vi "PFMate-Remote.vi"(2 "Channel":u8=1, 11 "Port":u8=1) -> ()   [LabVIEW 2009]
panel:
  in  "?":bool=TRUE
  in  "?":dbl(knob)=6.0 min=1.0 max=7.0 step=1.0 scale=1.0..7.0
  in  "?":dbl(knob)=5.0 min=1.0 max=7.0 step=1.0 scale=1.0..7.0
  in  "?":u8(ring)
  in  "?":u8(ring) items=["Run", "Float", "Brake"]
  in  "?":u8(ring) items=["Run", "Float", "Brake"]
  in  "?":bool=TRUE
  in  "PFMate address":u8=72 caption="PFMate Address" format="%x"
  # "Motor A"
  # "Motor B"
  # "mindsensors.com\nCopyright (c) 2009 by mindsensors.com\nEmail: info (<at>) mindsensors (<dot>) com\n\nThis program is free software. You can redistribute it and/or modify\nit under the terms of the GNU General Public License as published by\nthe Free Software Foundation; version 3 of the License.\nRead the license at: http://www.gnu.org/licenses/gpl.txt"
  # "Mode"
  # "Direction"
  # "Power"
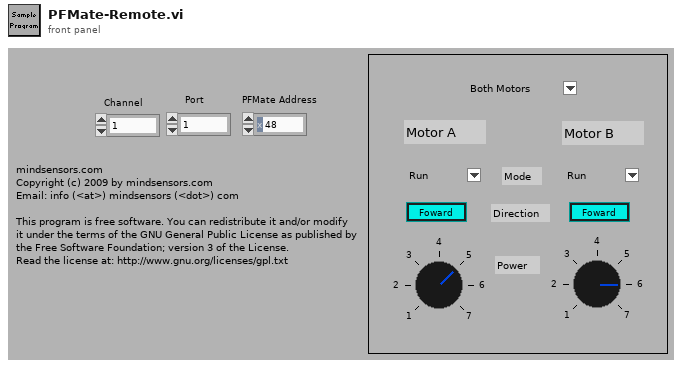
[diagram p1: front panel]
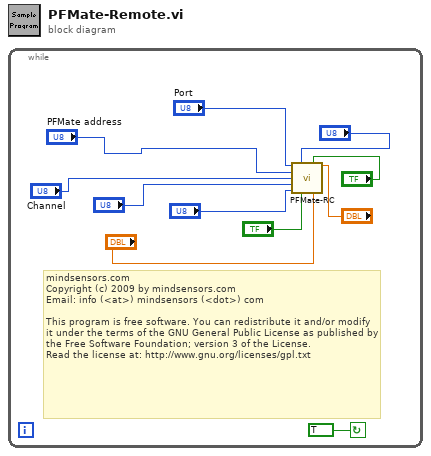
[diagram p0: block diagram]
diagram:
  n1 = while {
    stop <- TRUE continue-if-true
    # "mindsensors.com\nCopyright (c) 2009 by mindsensors.com\nEmail: info (<at>) mindsensors (<dot>) com\n\nThis program is free software. You can redistribute it and/or modify\nit under the terms of the GNU General Public License as published by\nthe Free Software Foundation; version 3 of the License.\nRead the license at: http://www.gnu.org/licenses/gpl.txt"
    n2 = call "PFMate-RC.vi"("Connection"="Port", "ModeB"="?", "DirectionB"="?", "PowerB"="?", "PFMate address"="PFMate address", "Channel"="Channel", "Operate_on"="?", "ModeA"="?", "DirectionA"="?", "PowerA"="?") -> ()  [unwired: 5 in, 1 out]
  }
